vi "Actividad1.vi"() -> ()   [LabVIEW 2026]
uses:
  <vilib>/Instr/_visa.llb/VISA Configure Serial Port (Instr).vi
panel:
  out "Indicador":string
  in  "VISA resource name":refnum<visa-resource-name>
  out "POT1":dbl(knob) scale=0.0..1023.0
  out "POT 2":dbl(knob) scale=0.0..1023.0
  out "POT 3":dbl(knob) scale=0.0..1023.0
  in  "ROJO":i64(knob) caption="A4" scale=0.0..255.0
  in  "A5":i64(knob) scale=0.0..255.0
  in  "A3":i64(knob) scale=0.0..255.0
  in  "LED 1":bool
  in  "LED 2":bool
  in  "LED 3":bool
  out "BOTON 3":bool
  out "BOTON 2":bool
  out "BOTON 1":bool
  in  "stop":bool
  out "Data Flow IN":string
  out "Data Flow OUT":string
  out "A3 Analog In temperatura":dbl(slide) scale=0.0..40.0
  out "Temperatura":dbl
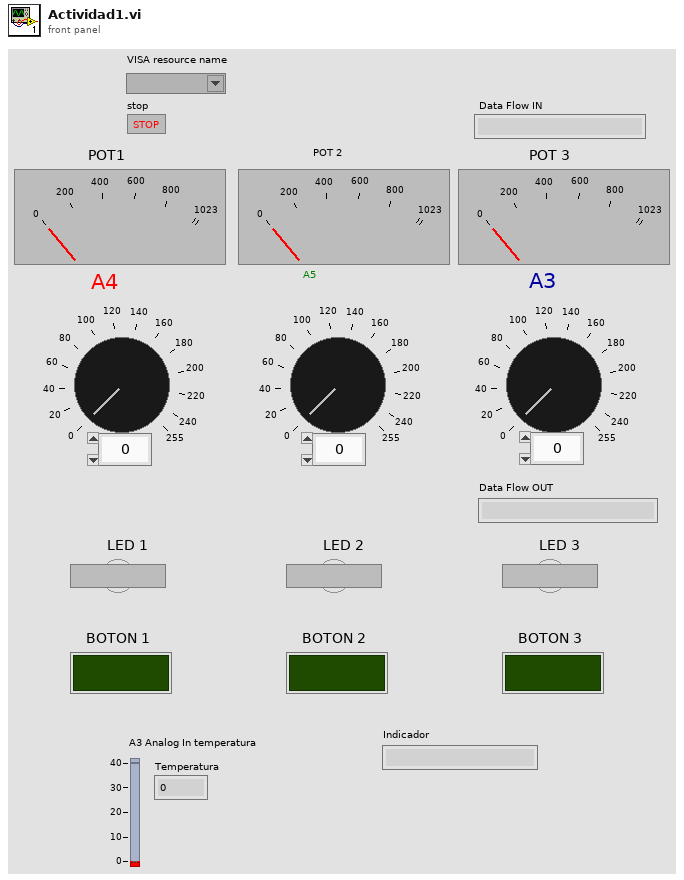
[diagram p1: front panel]
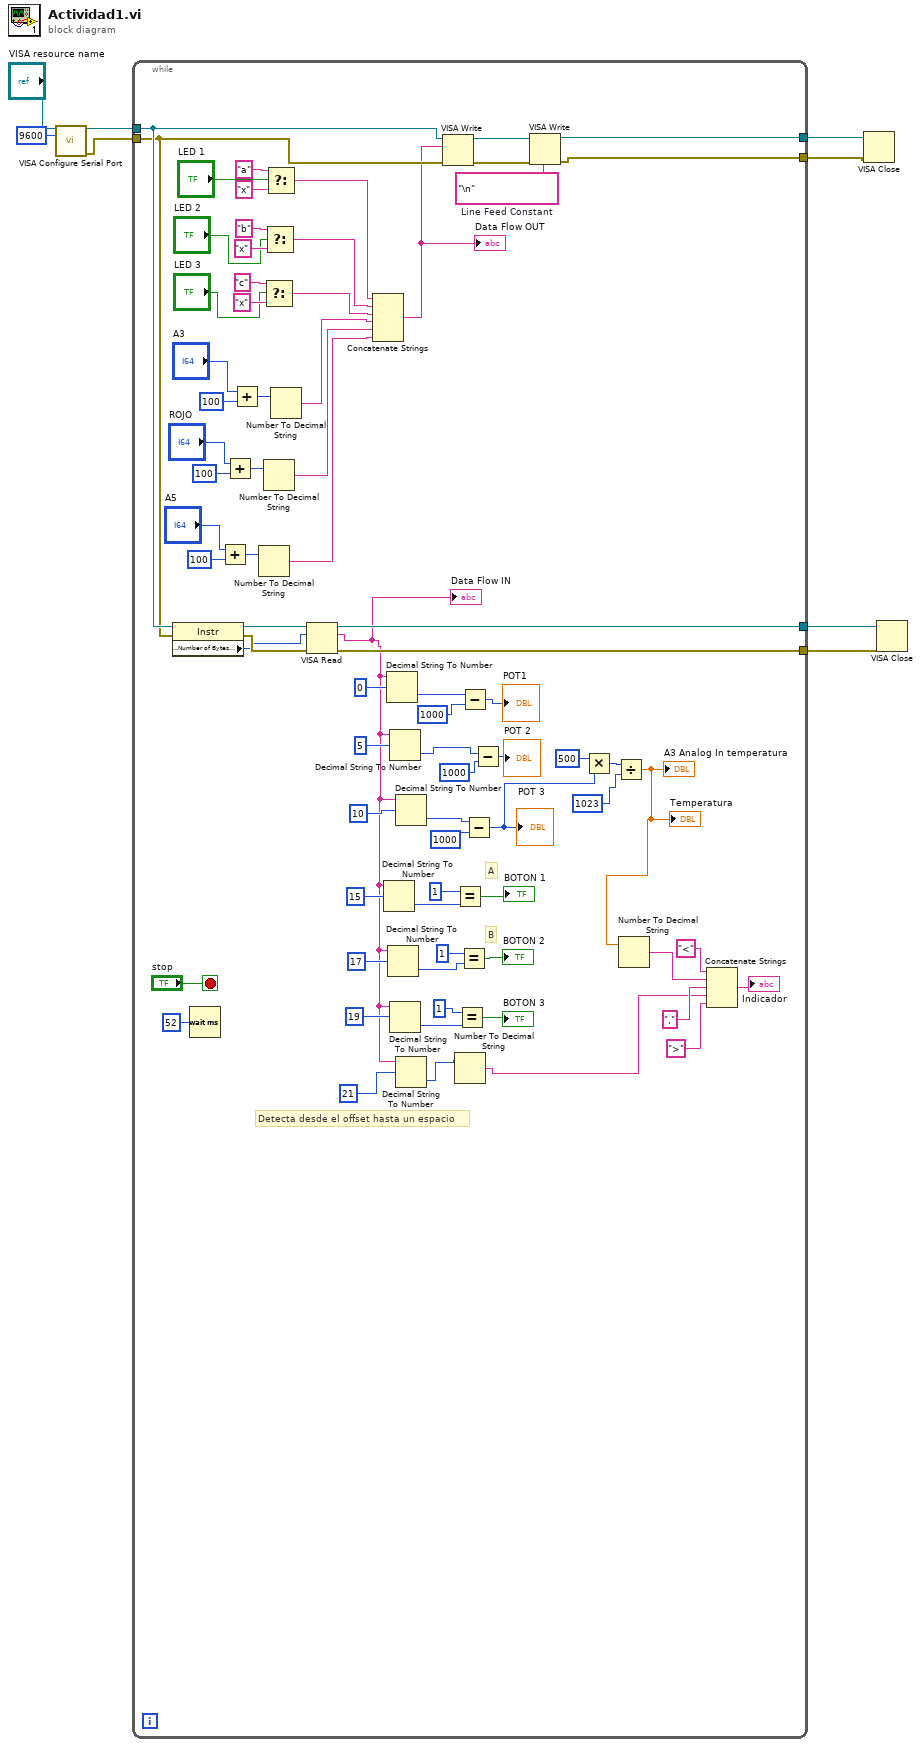
[diagram p0: block diagram]
diagram:
  n1 = call-poly "VISA Configure Serial Port"("VISA resource name"="VISA resource name", "baud rate (9600)"=u32 9600) -> ("VISA resource name out"=w8:refnum<visa-resource-name>, "error out"=w7:errorcluster)  [unwired: 12 in]
  n2 = while {
    tunnel: w8 -> [w39]
    tunnel: w7 -> [w38]
    tunnel: [w28] -> w4
    tunnel: [w43] -> w3
    tunnel: [w42] -> w2
    tunnel: [w41] -> w1
    stop <- "stop" stop-if-true
    w59 = "\n"  # Line Feed Constant
    # "Detecta desde el offset hasta un espacio"
    # "B"
    # "A"
    # "\\n"
    n3 = property class="Instr"(reference=w39, error in=w38) -> (reference out=w84:refnum<visa-resource-name>, error out=w83:errorcluster, "Serial Settings:Number of Bytes at Serial Port"=w82:u32)
    n4 = Wait (ms)(milliseconds to wait=u32 52) -> ()  [unwired: 1 out]
    n5 = Add(x="A5", y=i64 100) -> (x+y=w71:i64)
    n6 = Add(x="ROJO", y=i64 100) -> (x+y=w73:i64)
    n7 = Add(x="A3", y=i64 100) -> (x+y=w77:i64)
    n8 = Number To Decimal String(number=w71) -> (decimal integer string=w44:string)  [unwired: 1 in]
    n9 = Select(t="c", s="LED 3", f="x") -> (s? t:f=w47:string)
    n10 = Number To Decimal String(number=w73) -> (decimal integer string=w45:string)  [unwired: 1 in]
    n11 = Select(t="b", s="LED 2", f="x") -> (s? t:f=w48:string)
    n12 = Select(t="a", s="LED 1", f="x") -> (s? t:f=w57:string)
    n13 = Number To Decimal String(number=w77) -> (decimal integer string=w46:string)  [unwired: 1 in]
    n14 = VISA Read(VISA resource name=w84, byte count=w82, error in (no error)=w83) -> (VISA resource name out=w42:refnum<visa-resource-name>, read buffer=w15:string, error out=w41:errorcluster)  [unwired: 1 out]
    "Data Flow IN" <- w15
    n15 = Concatenate Strings "Concatenate Strings"(w57, w48, w47, w46, w45, w44) -> (w26:string)
    "Data Flow OUT" <- w26
    n16 = Decimal String To Number(string=w15, offset=15 ("offset (0)")) -> (number=w35:i32)  [unwired: 1 in, 1 out]
    n17 = Decimal String To Number(string=w15, offset=0) -> (number=w67:i32)  [unwired: 1 in, 1 out]
    n18 = Decimal String To Number(string=w15, offset=17 ("offset (0)")) -> (number=w31:i32)  [unwired: 1 in, 1 out]
    n19 = Decimal String To Number(string=w15, offset=5) -> (number=w63:i32)  [unwired: 1 in, 1 out]
    n20 = Decimal String To Number(string=w15, offset=19 ("offset (0)")) -> (number=w18:i32)  [unwired: 1 in, 1 out]
    n21 = Decimal String To Number(string=w15, offset=10) -> (number=w61:i32)  [unwired: 1 in, 1 out]
    n22 = Decimal String To Number(string=w15, offset=21) -> (number=w13:i32)  [unwired: 1 in, 1 out]
    n23 = VISA Write(VISA resource name=w39, write buffer=w26, error in (no error)=w38) -> (VISA resource name out=w27:refnum<visa-resource-name>, error out=w60:errorcluster)  [unwired: 1 out]
    n24 = Equal?(x=1 ("y"), y=w35) -> (x = y?=→"BOTON 1":bool)
    n25 = Number To Decimal String(number=w13) -> (decimal integer string=w9:string)  [unwired: 1 in]
    n26 = Equal?(x=1 ("y"), y=w18) -> (x = y?=→"BOTON 3":bool)
    n27 = Equal?(x=1 ("y"), y=w31) -> (x = y?=→"BOTON 2":bool)
    n28 = Subtract(x=w67, y=1000) -> (x-y=→"POT1":i32)
    n29 = Subtract(x=w61, y=1000) -> (x-y=w24:i32)
    "POT 3" <- w24
    n30 = Subtract(x=w63, y=1000) -> (x-y=→"POT 2":i32)
    n31 = VISA Write(VISA resource name=w27, write buffer=w59, error in (no error)=w60) -> (VISA resource name out=w28:refnum<visa-resource-name>, error out=w43:errorcluster)  [unwired: 1 out]
    n32 = Multiply(x=500, y=w24) -> (x*y=w23:i32)
    n33 = Divide(x=w23, y=1023) -> (x/y=w19:dbl)
    "A3 Analog In temperatura" <- w19
    "Temperatura" <- w19
    n34 = Number To Decimal String(number=w19) -> (decimal integer string=w17:string)  [unwired: 1 in]
    n35 = Concatenate Strings("<", w17, ",", w9, ">") -> (→"Indicador":string)
  }
  n36 = VISA Close(VISA resource name=w4, error in (no error)=w3) -> ()  [unwired: 1 out]
  n37 = VISA Close(VISA resource name=w2, error in (no error)=w1) -> ()  [unwired: 1 out]
